vi "CSM - Mark All Temp Variables as Permanent.vi"(8 "error in (no error)":errorcluster, 9 "Path (\"\" to Use Default File)":path) -> (2 "error out":errorcluster)   [LabVIEW 2017, in "INI-Static-Variable-Support.lvlib"]
uses:
  INI-Static-Variable-Support.lvlib
  _Support/_fgv-oper.ctl
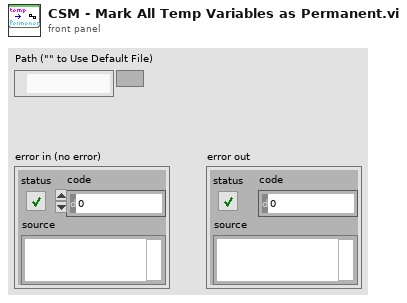
[diagram p1: front panel]
types:
  T1 = typedef "INI-Static-Variable-Support.lvlib/_fgv-oper.ctl" = enum16{"Read", "Write", "Sync", "Sessions", "List Keys", "Load", "List Files", "List Variables", "List Permanent Variables", "Mark Temp Variable as Permenent", "unload", "INIConfig(Memory)", "Reset", "Restore Variable Value"}
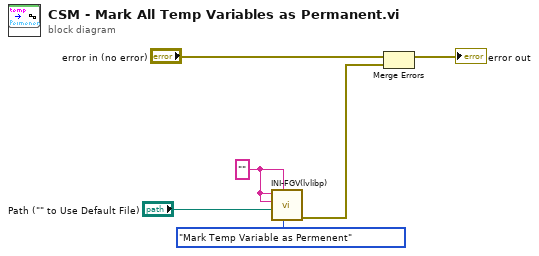
[diagram p0: block diagram]
diagram:
  w1 = "" (">> Variable Name >>")
  n1 = call "INI-FGV(lvlibp).vi"("Enum"=_fgv-oper."Mark Temp Variable as Permenent", "Prefered Section"=w1, "Path"="Path (\"\" to Use Default File)", ">> Default Value >>"=w1, ">> Variable Name >>"=w1) -> ("error out"=w4:errorcluster)  [unwired: 3 in, 3 out]
  n2 = Merge Errors("error in (no error)", w4) -> (→"error out":errorcluster)
